vi "ScaleData.vi"   [LabVIEW 2015]
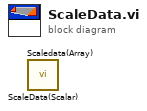
[diagram p0: block diagram]
diagram:
  n1 = call "ScaleData(Scalar).vi"() -> ()  [unwired: 11 in, 1 out]
  n2 = call "Scaledata(Array).vi"() -> ()  [unwired: 11 in, 1 out]
